vi "Configure Math (FFT).vi"(0 "VISA resource name":refnum<visa-resource-name>, 1 "Vertical Scale (2)":dbl=2.0, 2 "Vertical Offset (0)":dbl, 5 "Display Mode":enum16{"dBm", "Vrms", "Ampl", "PSD"}(ring), 7 "Horizontal Offset (0)":dbl, 9 "Horizontal scale":dbl, 11 "error in (no error)":errorcluster, 12 "Signal Source (1: Channel 1)":i32(ring)=1 items=["Channel 1"=1, "Channel 2"=2, "Channel 3"=3, "Channel 4"=4], 13 "Window Function (0: Rectangle)":i32(ring) items=["Rectangle", "Hanning", "Hamming", "Blackman"]) -> (4 "VISA resource name out":refnum<visa-resource-name>, 15 "error out":errorcluster)   [LabVIEW 2015, in "ZhiYuan ZDS Series for TCP.lvlib"]
doc: "Configures the setting for FFT math."
uses:
  ZhiYuan ZDS Series for TCP.lvlib
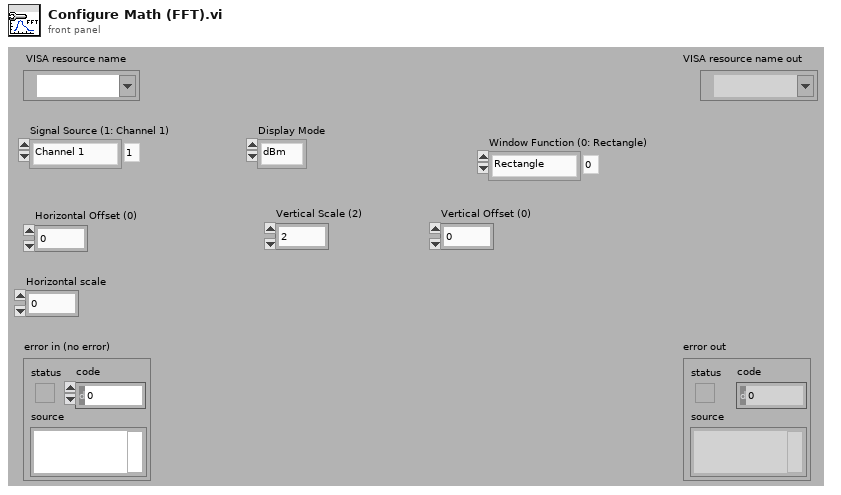
[diagram p1: front panel]
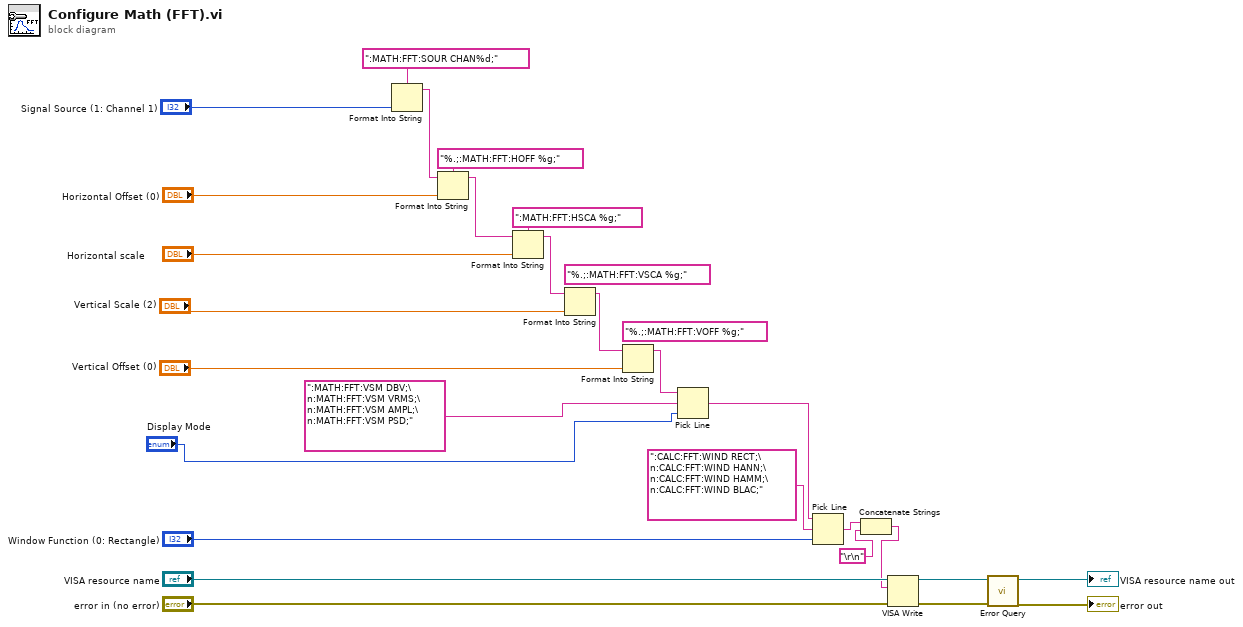
[diagram p0: block diagram]
diagram:
  (unwired) "%.;:MATH:FFT:VOFF %g;"
  (unwired) "%.;:MATH:FFT:VSCA %g;"
  n1 = Format Into String(format string=":MATH:FFT:SOUR CHAN%d;", "Signal Source (1: Channel 1)") -> (resulting string=w12:string)  [unwired: 2 in, 1 out]
  n2 = Format Into String(format string="%.;:MATH:FFT:HOFF %g;", initial string=w12, "Horizontal Offset (0)") -> (resulting string=w25:string)  [unwired: 1 in, 1 out]
  n3 = Format Into String(format string=":MATH:FFT:HSCA %g;", initial string=w25, "Horizontal scale") -> (resulting string=w9:string)  [unwired: 1 in, 1 out]
  n4 = Format Into String(initial string=w9, "Vertical Scale (2)") -> (resulting string=w8:string)  [unwired: 2 in, 1 out]
  n5 = Format Into String(initial string=w8, "Vertical Offset (0)") -> (resulting string=w7:string)  [unwired: 2 in, 1 out]
  n6 = Pick Line(string ("")=w7, multi-line string=":MATH:FFT:VSM DBV;\n:MATH:FFT:VSM VRMS;\n:MATH:FFT:VSM AMPL;\n:MATH:FFT:VSM PSD;", line index="Display Mode") -> (output string=w4:string)
  n7 = Pick Line(string ("")=w4, multi-line string=":CALC:FFT:WIND RECT;\n:CALC:FFT:WIND HANN;\n:CALC:FFT:WIND HAMM;\n:CALC:FFT:WIND BLAC;", line index="Window Function (0: Rectangle)") -> (output string=w3:string)
  n8 = Concatenate Strings(w3, "\r\n") -> (w1:string)
  n9 = VISA Write(VISA resource name="VISA resource name", write buffer=w1, error in (no error)="error in (no error)") -> (VISA resource name out=w17:refnum<visa-resource-name>, error out=w16:errorcluster)  [unwired: 1 out]
  n10 = call "Error Query.vi"("error in (no error)"=w16, "VISA resource name"=w17) -> ("error out"=→"error out":errorcluster, "VISA resource name out"=→"VISA resource name out":refnum<visa-resource-name>)  [unwired: 6 in, 2 out]
